vi "reset_pattern.vi"(8 "error in (no error)":errorcluster, 11 "StimulatorDL090503 in":refnum<class "StimulatorDL090503.lvclass">) -> (0 "error out":errorcluster, 3 "StimulatorDL090503 out":refnum<class "StimulatorDL090503.lvclass">)   [LabVIEW 2010, in "StimulatorDL090503.lvclass"]
uses:
  StimulatorDL090503.lvclass
  common/enumerations/functional_global_action_enum.ctl
  StimulatorDL090503.lvclass/StimulatorDL090503.ctl
  SignalWriter/GenericSignalWriter/GenericSignalWriter/GenericSignalWriter.lvclass
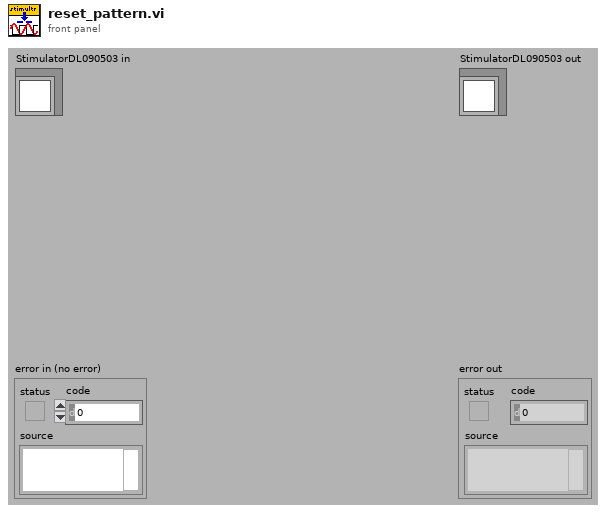
[diagram p1: front panel]
types:
  T1 = typedef "functional_global_action_enum.ctl" = enum16{"get", "set", "reset"}
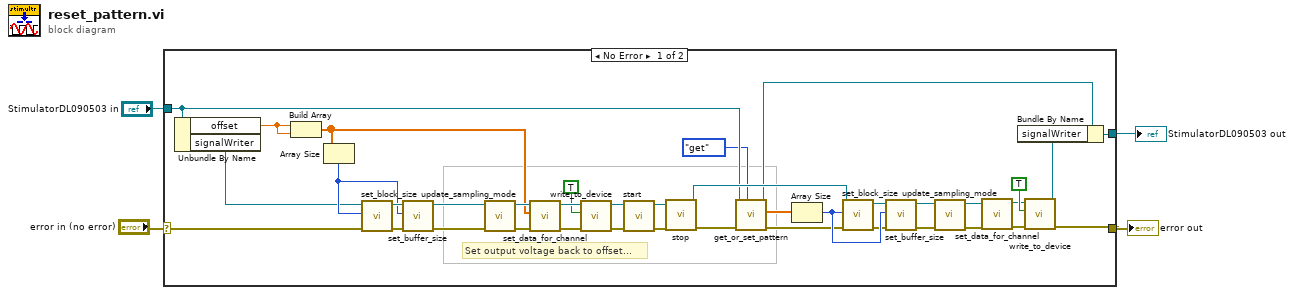
[diagram p0: block diagram]
diagram:
  n1 = case shown="No Error" "error in (no error)" {
    selector: "error in (no error)" -> [w30 w44]
    tunnel: [w15 w44] -> w1
    tunnel: [w27 w43] -> w2
    tunnel: "StimulatorDL090503 in" -> [w9 w43]
    frame No Error {
      # "Set output voltage back to offset..."
      n2 = Unbundle By Name(w9) -> ("offset"=w14:dbl, "signalWriter"=w29:refnum<class "GenericSignalWriter.lvclass">)
      n3 = Build Array(w14, w14) -> (w28:dbl[])
      n4 = Array Size(array=w28) -> (size(s)=w31:i32)
      n5 = call "set_block_size.vi"("error in (no error)"=w30, "block size (samples)"=w31, "GenericWriteSignals.lvclass in"=w29) -> ("error out"=w34:errorcluster, "GenericWriteSignals.lvclass out"=w35:refnum<class "GenericSignalWriter.lvclass">)  [unwired: 7 in]
      n6 = call-dynamic "set_buffer_size.vi"("error in (no error)"=w34, "buffer size (samples)"=w31, "GenericWriteSignals.lvclass in"=w35) -> ("error out"=w13:errorcluster, "GenericWriteSignals.lvclass out"=w12:refnum<class "GenericSignalWriter.lvclass">)  [unwired: 7 in]
      n7 = call-dynamic "update_sampling_mode.vi"("error in (no error)"=w13, "GenericWriteSignals in"=w12) -> ("error out"=w33:errorcluster, "GenericWriteSignals out"=w32:refnum<class "GenericSignalWriter.lvclass">)  [unwired: 8 out]
      n8 = call-dynamic "set_data_for_channel.vi"("error in (no error)"=w33, "data"=w28, "GenericWriteSignals in"=w32) -> ("error out"=w41:errorcluster, "GenericWriteSignals out"=w42:refnum<class "GenericSignalWriter.lvclass">)  [unwired: 7 out]
      n9 = call-dynamic "write_to_device.vi"("error in (no error)"=w41, "force writing?"=TRUE, "GenericWriteSignals in"=w42) -> ("error out"=w39:errorcluster, "GenericWriteSignals out"=w38:refnum<class "GenericSignalWriter.lvclass">)  [unwired: 7 out]
      n10 = call-dynamic "start.vi"("error in (no error)"=w39, "WriteSignalsGenericPlugin in"=w38) -> ("error out"=w37:errorcluster, "WriteSignalsGenericPlugin out"=w36:refnum<class "GenericSignalWriter.lvclass">)  [unwired: 8 out]
      n11 = call-dynamic "stop.vi"("error in (no error)"=w37, "WriteSignalsGenericPlugin in"=w36) -> ("error out"=w11:errorcluster, "WriteSignalsGenericPlugin out"=w21:refnum<class "GenericSignalWriter.lvclass">)  [unwired: 8 out]
      n12 = call "get_or_set_pattern.vi"("action"=functional_global_action_enum."get", "error in (no error)"=w11, "StimulatorDL090503 in"=w9) -> ("error out"=w10:errorcluster, "pattern out"=w6:dbl[], "StimulatorDL090503 out"=w8:refnum<class "StimulatorDL090503.lvclass">)  [unwired: 6 in]
      n13 = Array Size(array=w6) -> (size(s)=w26:i32)
      n14 = call "set_block_size.vi"("error in (no error)"=w10, "block size (samples)"=w26, "GenericWriteSignals.lvclass in"=w21) -> ("error out"=w25:errorcluster, "GenericWriteSignals.lvclass out"=w22:refnum<class "GenericSignalWriter.lvclass">)  [unwired: 7 in]
      n15 = call-dynamic "set_buffer_size.vi"("error in (no error)"=w25, "buffer size (samples)"=w26, "GenericWriteSignals.lvclass in"=w22) -> ("error out"=w24:errorcluster, "GenericWriteSignals.lvclass out"=w23:refnum<class "GenericSignalWriter.lvclass">)  [unwired: 7 in]
      n16 = call-dynamic "update_sampling_mode.vi"("error in (no error)"=w24, "GenericWriteSignals in"=w23) -> ("error out"=w17:errorcluster, "GenericWriteSignals out"=w16:refnum<class "GenericSignalWriter.lvclass">)  [unwired: 8 out]
      n17 = call-dynamic "set_data_for_channel.vi"("error in (no error)"=w17, "GenericWriteSignals in"=w16) -> ("error out"=w19:errorcluster, "GenericWriteSignals out"=w18:refnum<class "GenericSignalWriter.lvclass">)  [unwired: 1 in, 7 out]
      n18 = call-dynamic "write_to_device.vi"("error in (no error)"=w19, "force writing?"=TRUE, "GenericWriteSignals in"=w18) -> ("error out"=w15:errorcluster, "GenericWriteSignals out"=w5:refnum<class "GenericSignalWriter.lvclass">)  [unwired: 7 out]
      n19 = Bundle By Name(cluster=w8, "signalWriter"=w5) -> (w27:refnum<class "StimulatorDL090503.lvclass">)
    }
    frame Error {
    }
  }
  "error out" <- w1
  "StimulatorDL090503 out" <- w2
